vi "用户确认数据.vi"(9 "WIFI NAME":string caption="请打开无线界面刷新确认有以下名称的WIFI热点") -> (2 "result":bool)   [LabVIEW 2013]
panel:
  in  "fail":bool
  in  "pass":bool
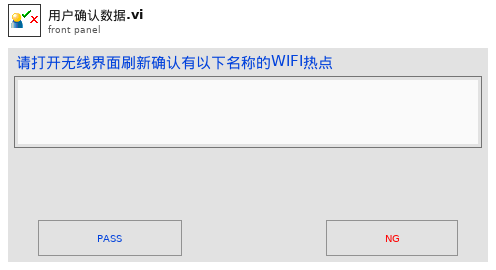
[diagram p1: front panel]
types:
  T1 = enum8{"Enabled", "Disabled", "Disabled and Grayed Out"}
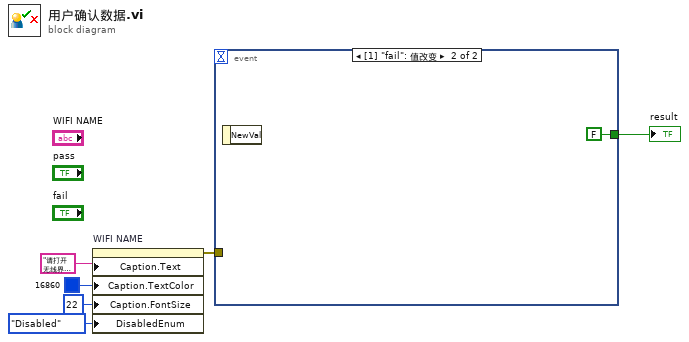
[diagram p0: block diagram]
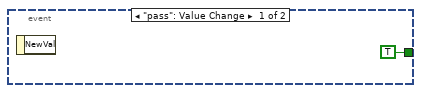
[diagram p2: hidden frame]
diagram:
  n1 = property on="WIFI NAME" class="Str"("Caption.Text"="请打开无线界面刷新确认有以下名称的WIFI热点" ("提示"), "Caption.TextColor"=u32 16860, "Caption.FontSize"=u32 22 ("标题.字体:字号"), "DisabledEnum"=T1."Disabled" ("禁用")) -> (error out=w3:errorcluster)  [unwired: 2 in, 1 out]
  n2 = event shown="[1] \"fail\": 值改变" {
    selector: _ -> [_ _]
    dyn-events: _ -> [_ _]
    timeout: _ -> [_ _]
    tunnel: w3 -> [_ _]
    tunnel: [TRUE ("NewVal") FALSE ("NewVal")] -> w2
    event "pass": Value Change {
      n3 = event-data() -> ()  [unwired: 1 in, 1 out]
    }
    event "fail": Value Change {
      n4 = event-data() -> ()  [unwired: 1 in, 1 out]
    }
  }
  "result" <- w2
